vi "UltrasonicGetValue.vi"() -> (3 "ultrasonicValue":dbl)   [LabVIEW 2014]
uses:
  ultrasonicGlobal.vi
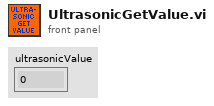
[diagram p1: front panel]
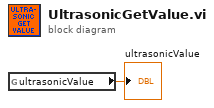
[diagram p0: block diagram]
diagram:
  n1 = global read "ultrasonicGlobal.vi" "ultrasonicValue"() -> (→"ultrasonicValue":dbl)
